vi "TimerbNN.vi"(11 "stop":bool) -> (0 "Sumarized":dbl format="%#_2g", 3 "Time s":dbl format="%#_2g")   [LabVIEW 2023]
panel:
  out "Reset":bool
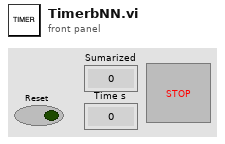
[diagram p1: front panel]
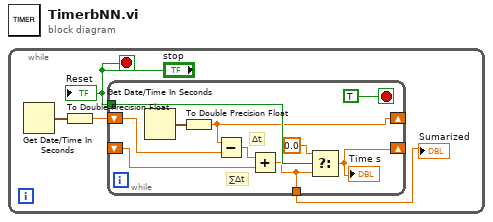
[diagram p0: block diagram]
diagram:
  n1 = while {
    stop <- "stop" stop-if-true
    n2 = Get Date/Time In Seconds() -> (seconds since 1Jan1904=w3:timestamp)
    n3 = To Double Precision Float(number=w3) -> (double precision float=w2:dbl)
    n4 = while {
      shift-right: [w8] -> _
      shift-left: _ -> [w11]
      tunnel: "stop" -> [w10]
      shift-right: [w7] -> _
      shift-left: w2 -> [w13]
      tunnel: [w6] -> w4
      stop <- TRUE stop-if-true
      # "∑∆t"
      # "∆t"
      n5 = Get Date/Time In Seconds() -> (seconds since 1Jan1904=w14:timestamp)
      n6 = To Double Precision Float(number=w14) -> (double precision float=w7:dbl)
      n7 = Subtract(x=w7, y=w13) -> (x-y=w12:dbl)
      n8 = Add(x=w12, y=w11) -> (x+y=w6:dbl)
      n9 = Select(t=0.0, s=w10, f=w6) -> (s? t:f=w8:dbl)
      "Time s" <- w8
    }
    "Sumarized" <- w4
    "Reset" <- "stop"
  }
